vi "Punto 2 _ JUAN BERMUDEZ.vi"() -> ()   [LabVIEW 2020]
panel:
  in  "stop":bool
  out "Vocales segunda mitad":i32
  out "Vocales primera mitad":i32
  out "Vocales totales, para resultado correcto, recuerde refrescar":i32
  in  "Accionar":bool
  out "Segunda mitad":string
  out "Primera mitad":string
  in  "Textro inicial":string
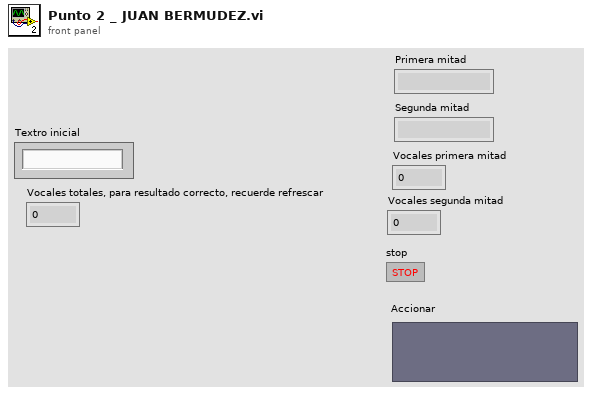
[diagram p1: front panel]
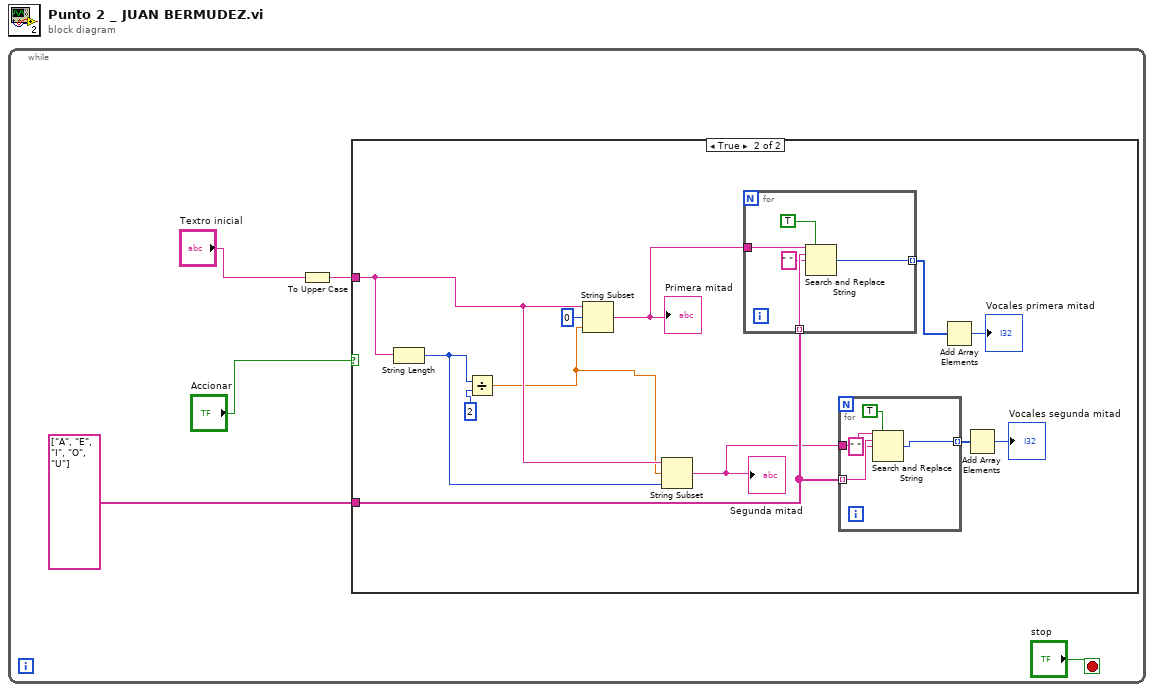
[diagram p0: block diagram]
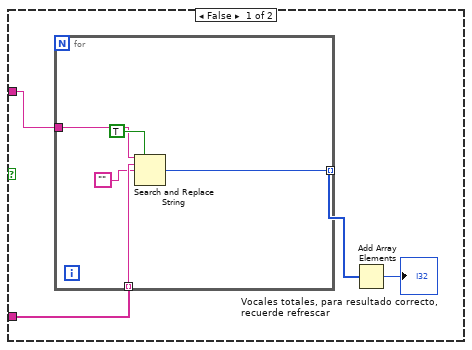
[diagram p2: hidden frame]
diagram:
  n1 = while {
    stop <- "stop" stop-if-true
    n2 = To Upper Case(1:"Textro inicial") -> (0:w5:string)
    n3 = case shown="True" "Accionar" {
      tunnel: w5 -> [w9 w24]
      tunnel: string[] ["A", "E", "I", "O", "U"] -> [w8 w20]
      frame False {
        n4 = for {
          tunnel: w9 -> [w10]
          tunnel: w8 -> [w14] mode=indexing
          tunnel: [w12] -> w7 mode=indexing
          n5 = Search and Replace String(replace all?=TRUE ("replace all? (F)"), input string=w10, search string=w14, replace string="") -> (number of replacements=w12:i32)  [unwired: 4 in, 3 out]
        }
        n6 = Add Array Elements(numeric array=w7) -> (sum=→"Vocales totales, para resultado correcto, recuerde refrescar":i32)
      }
      frame True {
        n7 = String Length(string=w24) -> (length=w23:i32)
        n8 = Divide(x=w23, y=2) -> (x/y=w17:dbl)
        n9 = String Subset(string=w24, offset (0)=0, length (rest)=w17) -> (substring=w16:string)
        "Primera mitad" <- w16
        n10 = String Subset(string=w24, offset (0)=w17, length (rest)=w23) -> (substring=w15:string)
        "Segunda mitad" <- w15
        n11 = for {
          tunnel: w20 -> [w36] mode=indexing
          tunnel: [w35] -> w22 mode=indexing
          tunnel: w16 -> [w34]
          n12 = Search and Replace String(replace all?=TRUE ("replace all? (F)"), input string=w34, search string=w36, replace string=" " ("replace string (\"\")")) -> (number of replacements=w35:i32)  [unwired: 4 in, 3 out]
        }
        n13 = for {
          tunnel: w20 -> [w31] mode=indexing
          tunnel: [w30] -> w18 mode=indexing
          tunnel: w15 -> [w29]
          n14 = Search and Replace String(replace all?=TRUE ("replace all? (F)"), input string=w29, search string=w31, replace string=" " ("replace string (\"\")")) -> (number of replacements=w30:i32)  [unwired: 4 in, 3 out]
        }
        n15 = Add Array Elements(numeric array=w22) -> (sum=→"Vocales primera mitad":i32)
        n16 = Add Array Elements(numeric array=w18) -> (sum=→"Vocales segunda mitad":i32)
      }
    }
  }
